vi "Easy XML AND DotNET Signature.vi"() -> ()   [LabVIEW 2016]
panel:
  out "error out":errorcluster
  in  "error in (no error)":errorcluster
  out "Signed XML String":string
  in  "Data to Sign":T1={"Data To Secure"={"Critical Data"={"Data to protect"="Important Data", "More data to protect"="More Important Data"}}}
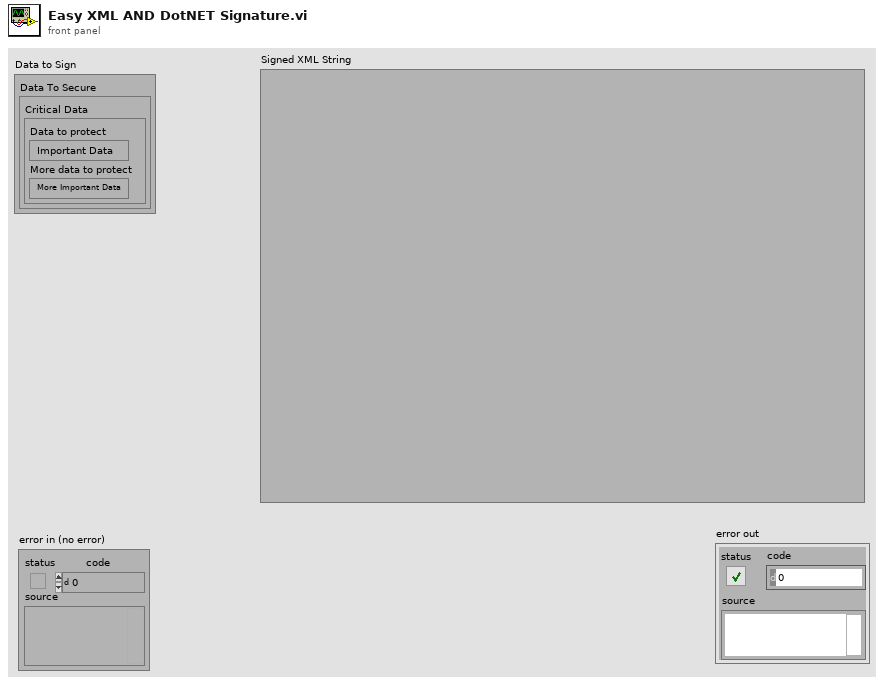
[diagram p1: front panel]
types:
  T1 = cluster{"Data To Secure":cluster{"Critical Data":cluster{"Data to protect":string, "More data to protect":string}}}
  T2 = cluster{"Critical Data":cluster{"Data to protect":string, "More data to protect":string}}
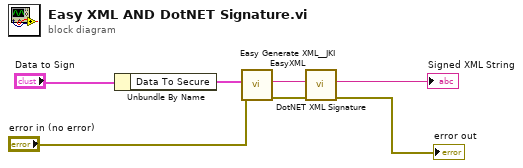
[diagram p0: block diagram]
diagram:
  n1 = Unbundle By Name("Data to Sign") -> ("Data To Secure"=w7:T2)
  n2 = call <vilib>:"Easy Generate XML__JKI EasyXML.vi"("error in (no error)"="error in (no error)", "LabVIEW Data"=w7) -> ("error out"=w4:errorcluster, "XML String"=w5:string)  [unwired: 8 in]
  n3 = call "DotNET XML Signature.vi"("error in (no error)"=w4, "XML String In"=w5) -> ("error out"=→"error out":errorcluster, "Signed XML"=→"Signed XML String":string)  [unwired: 8 in]
